vi "iHR550 Set Values.vi"(0 "Refnum out":refnum<k7>, 1 "Entrance Mirror":u16(ring)=2 caption="Target Position\nEntrance Mirror" items=["Front"=2, "Side"=3], 3 "Target\nSide Entrance":dbl, 5 "iHR Settings":T1={"iHR550 Set Exit Mirror"=2, "iHR550 Set Side Exit"=0.0, "iHR550 Set Front Entrance"=0.0, "iHR550 Set Wavelength"=897.9988, "iHR550 Set Grating"=0, "iHR550 Set Grating Switch"=FALSE, "iHR550 Set Wavelength Switch"=FALSE, "iHR550 Set Mirror Switch"=FALSE, "iHR550 Set Slits Switch"=FALSE} {"iHR550 Set Wavelength" min=0.0 max=1500.0 step=1.0; "iHR550 Set Side Exit" min=0.0 max=2000.0 step=1.0; "iHR550 Set Exit Mirror" items=["Front"=2, "Side"=3]}, 11 "error in (no error)":errorcluster, 13 "Target\nFront Exit":dbl) -> (15 "error out":errorcluster)   [LabVIEW 2010]
uses:
  TypeDefs/iHR Settings.ctl
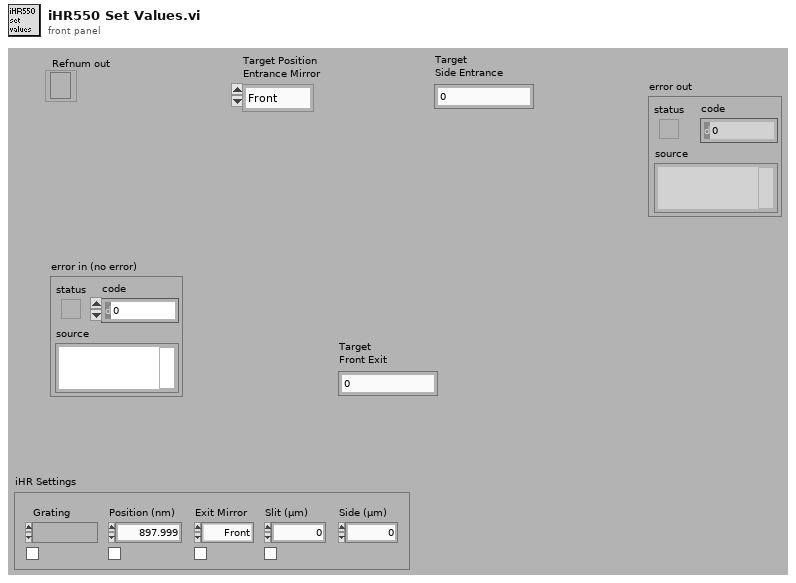
[diagram p1: front panel]
types:
  T1 = typedef "iHR Settings.ctl" = cluster{"iHR550 Set Exit Mirror":u16, "iHR550 Set Side Exit":dbl, "iHR550 Set Front Entrance":dbl, "iHR550 Set Wavelength":dbl, "iHR550 Set Grating":u16, "iHR550 Set Grating Switch":bool, "iHR550 Set Wavelength Switch":bool, "iHR550 Set Mirror Switch":bool, "iHR550 Set Slits Switch":bool}
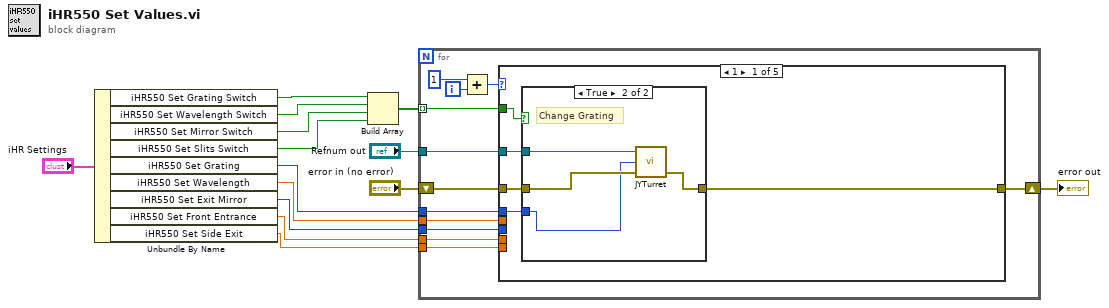
[diagram p0: block diagram]
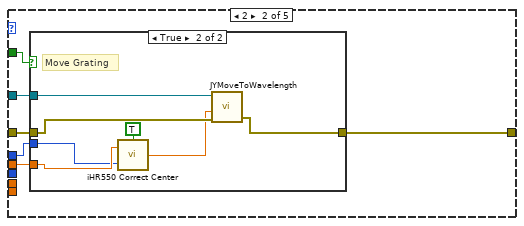
[diagram p3: hidden frame]
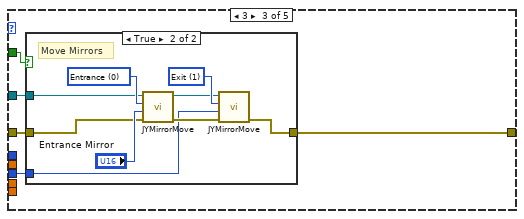
[diagram p5: hidden frame]
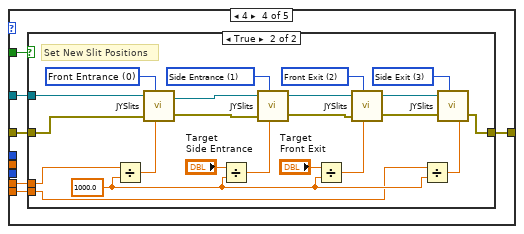
[diagram p7: hidden frame]
diagram:
  n1 = Unbundle By Name("iHR Settings") -> ("iHR550 Set Grating Switch"=w7:bool, "iHR550 Set Wavelength Switch"=w10:bool, "iHR550 Set Mirror Switch"=w9:bool, "iHR550 Set Slits Switch"=w8:bool, "iHR550 Set Grating"=w5:u16, "iHR550 Set Wavelength"=w4:dbl, "iHR550 Set Exit Mirror"=w3:u16, "iHR550 Set Front Entrance"=w2:dbl, "iHR550 Set Side Exit"=w1:dbl)
  n2 = Build Array(w7, w10, w9, w8) -> (w6:bool[])
  n3 = for {
    tunnel: w6 -> [w26] mode=indexing
    tunnel: "Refnum out" -> [w25]
    shift-right: [w24] -> w13
    shift-left: "error in (no error)" -> [w23]
    tunnel: w5 -> [w19]
    tunnel: w4 -> [w18]
    tunnel: w3 -> [w17]
    tunnel: w2 -> [w16]
    tunnel: w1 -> [w15]
    i -> [w22]
    n4 = Add(x=1, y=w22) -> (x+y=w20:i32)
    n5 = case shown="1" w20 {
      tunnel: w26 -> [w31 w39 w52 w71 _]
      tunnel: w25 -> [w30 w40 w53 w68 _]
      tunnel: [w29 w42 w54 w69 w95] -> w24
      tunnel: w23 -> [w28 w41 w55 w70 w95]
      tunnel: w19 -> [w27 w37 _ _ _]
      tunnel: w18 -> [_ w38 _ _ _]
      tunnel: w17 -> [_ _ w51 _ _]
      tunnel: w16 -> [_ _ _ w67 _]
      tunnel: w15 -> [_ _ _ w66 _]
      frame 1 {
        n6 = case shown="True" w31 {
          tunnel: w30 -> [_ w36]
          tunnel: [w32 w35] -> w29
          tunnel: w28 -> [w32 w34]
          tunnel: w27 -> [_ w33]
          frame False {
          }
          frame True {
            # "Change Grating"
            n7 = call "JYTurret.vi"("error in (no error)"=w34, "Grating Index"=w33, "JYMONOLib.IJYMonoReqd"=w36) -> ("error out"=w35:errorcluster)  [unwired: 2 out]
          }
        }
      }
      frame 2 {
        n8 = case shown="True" w39 {
          tunnel: w40 -> [_ w50]
          tunnel: w41 -> [w43 w49]
          tunnel: [w43 w48] -> w42
          tunnel: w38 -> [_ w47]
          tunnel: w37 -> [_ w44]
          frame False {
          }
          frame True {
            # "Move Grating"
            n9 = call "iHR550 Correct Center.vi"("Set?"=TRUE, "Grating Index"=w44, "Position In (nm)"=w47) -> ("Position Out (nm)"=w45:dbl)
            n10 = call "JYMoveToWavelength.vi"("error in (no error)"=w49, "Target WL"=w45, "RefNum In"=w50) -> ("error out"=w48:errorcluster)  [unwired: 1 in, 2 out]
          }
        }
      }
      frame 3 {
        n11 = case shown="True" w52 {
          tunnel: w55 -> [w56 w61]
          tunnel: [w56 w60] -> w54
          tunnel: w53 -> [_ w58]
          tunnel: w51 -> [_ w59]
          frame False {
          }
          frame True {
            w64 = u16 1 items=["Entrance", "Exit", "Front", "Side"] ("Mirror Number")
            w62 = u16 0 items=["Entrance", "Exit", "Front", "Side"] ("Mirror Number")
            # "Move Mirrors"
            n12 = call "JYMirrorMove.vi"("error in (no error)"=w61, "Mirror Position"="Entrance Mirror", "Mirror Number"=w62, "RefNum In"=w58) -> ("error out"=w65:errorcluster, "MonoRefNum Out"=w57:refnum<k7>)  [unwired: 6 in]
            n13 = call "JYMirrorMove.vi"("error in (no error)"=w65, "Mirror Position"=w59, "Mirror Number"=w64, "RefNum In"=w57) -> ("error out"=w60:errorcluster)  [unwired: 6 in, 1 out]
          }
        }
      }
      frame 4 {
        n14 = case shown="True" w71 {
          tunnel: w70 -> [w72 w84]
          tunnel: [w72 w82] -> w69
          tunnel: w68 -> [_ w83]
          tunnel: w67 -> [_ w74]
          tunnel: w66 -> [_ w73]
          frame False {
          }
          frame True {
            w81 = 1000.0 ("y")
            w94 = u16 3 items=["Front Entrance", "Side Entrance", "Front Exit", "Side Exit", "First Intermediate", "Second Intermediate"] ("Slit")
            w93 = u16 2 items=["Front Entrance", "Side Entrance", "Front Exit", "Side Exit", "First Intermediate", "Second Intermediate"] ("Slit")
            w92 = u16 1 items=["Front Entrance", "Side Entrance", "Front Exit", "Side Exit", "First Intermediate", "Second Intermediate"] ("Slit")
            w91 = u16 0 items=["Front Entrance", "Side Entrance", "Front Exit", "Side Exit", "First Intermediate", "Second Intermediate"] ("Slit")
            # "Set New Slit Positions"
            n15 = Divide(x=w74, y=w81) -> (x/y=w78:dbl)
            n16 = call "JYSlits.vi"("JYMONOLib.IJYMonoReqd"=w83, "Slit"=w91, "error in (no error)"=w84, "Slit Width"=w78) -> ("JYMONOLib.IJYMonoReqd 2"=w85:refnum<k7>, "error out"=w88:errorcluster)  [unwired: 1 in]
            n17 = Divide(x="Target\nSide Entrance", y=w81) -> (x/y=w77:dbl)
            n18 = call "JYSlits.vi"("JYMONOLib.IJYMonoReqd"=w85, "Slit"=w92, "error in (no error)"=w88, "Slit Width"=w77) -> ("JYMONOLib.IJYMonoReqd 2"=w86:refnum<k7>, "error out"=w89:errorcluster)  [unwired: 1 in]
            n19 = Divide(x="Target\nFront Exit", y=w81) -> (x/y=w76:dbl)
            n20 = call "JYSlits.vi"("JYMONOLib.IJYMonoReqd"=w86, "Slit"=w93, "error in (no error)"=w89, "Slit Width"=w76) -> ("JYMONOLib.IJYMonoReqd 2"=w87:refnum<k7>, "error out"=w90:errorcluster)  [unwired: 1 in]
            n21 = Divide(x=w73, y=w81) -> (x/y=w75:dbl)
            n22 = call "JYSlits.vi"("JYMONOLib.IJYMonoReqd"=w87, "Slit"=w94, "error in (no error)"=w90, "Slit Width"=w75) -> ("error out"=w82:errorcluster)  [unwired: 1 in, 1 out]
          }
        }
      }
      frame 5, Default {
      }
    }
  }
  "error out" <- w13
